vi "Open.vi"(8 "error in (no error)":errorcluster, 9 "name (unnamed)":string, 10 "max queue size (-1, unlimited)":i32=20) -> (0 "error out":errorcluster, 3 "queue out":refnum<queue>)   [LabVIEW 2019, in "Simple Queue Message.lvlib"]
uses:
  Simple Queue Message.lvlib
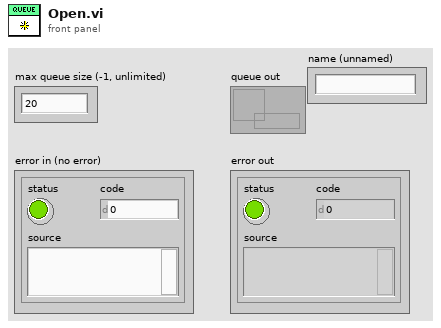
[diagram p1: front panel]
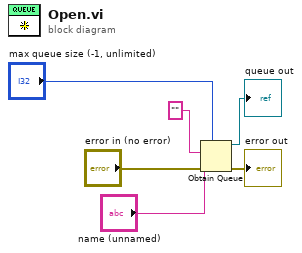
[diagram p0: block diagram]
diagram:
  n1 = Obtain Queue(max queue size (-1, unlimited)="max queue size (-1, unlimited)", name (unnamed)="name (unnamed)", element data type="", error in (no error)="error in (no error)") -> (queue out=→"queue out":refnum<queue>, error out=→"error out":errorcluster)  [unwired: 1 in, 1 out]
